vi "总磷氨氮插入数据.vi"(0 "database":string, 1 "data":T1 {"单位" items=["ug/L", "mg/L", "ppm", "mg/m3", "cm", "ppb", "ug/m3", "%", "nmol/mol", "umol/mol", "MPN/L", "MPN/100ml", "ng/m3", "NTU", "无量纲", "ms/cm", "us/cm"]}, 3 "SN":string, 5 "table":string, 7 "测量模式":T2(ring)=enum."水样测试", 9 "数据标记表":string(combo)="N", 11 "error in (no error)":errorcluster) -> (15 "error out":errorcluster)   [LabVIEW 2016, in "斯坦道氨氮.lvlib"]
uses:
  <vilib>/Utility/sysdir.llb/System Directory Type.ctl
  <vilib>/Utility/error.llb/DialogType.ctl
  <vilib>/addons/database/Connection.llb/DB Tools Open Connec (String).vi
  <vilib>/addons/database/Connection.llb/Conn Execute.vi
  <vilib>/addons/database/Recordset.llb/Rec Destroy - Connection.vi
  <vilib>/addons/database/Recordset.llb/Rec Fetch Recordset Data (R).vi
  <vilib>/addons/database/NI_Database_API.lvlib
panel:
  out "为空？":bool
  out "recordset data":variant[][](array[variant])
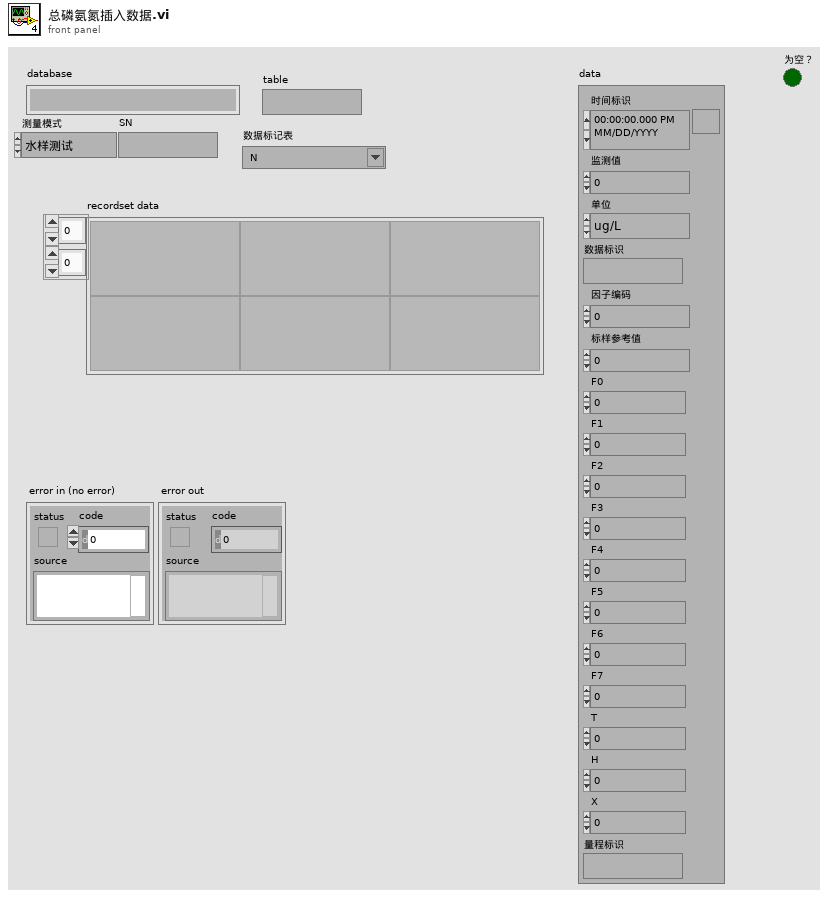
[diagram p1: front panel]
types:
  T1 = cluster{"时间标识":timestamp, "监测值":sgl, "单位":u16, "数据标识":string, "因子编码":u32, "标样参考值":sgl, "F0":sgl, "F1":sgl, "F2":sgl, "F3":sgl, "F4":sgl, "F5":sgl, "F6":sgl, "F7":sgl, "T":sgl, "H":sgl, "X":sgl, "量程标识":string}
  T2 = enum16{"维护数据", "水样测试", "标样核查", "零点核查", "跨度核查", "空白测试", "平行样测试", "加标回收", "空白校准", "标样校准", "初始化（清洗）"}
  T3 = typedef "DialogType.ctl" = u16
  T4 = typedef "System Directory Type.ctl" = i32
  T5 = typedef "NI_Database_API.lvlib/Conn ObjectReference.ctl" = refnum<k1>
  T6 = typedef "NI_Database_API.lvlib/Rec ObjectReference.ctl" = refnum<k1>
  T7 = cluster{"时间标识":timestamp, "测量模式":string, "数据类型":string, "监测值":sgl, "单位":string, "数据标识":string, "因子编码":string, "标样参考值":sgl, "F0":sgl, "F1":sgl, "F2":sgl, "F3":sgl, "F4":sgl, "F5":sgl, "F6":sgl, "F7":sgl, "温度":sgl, "湿度":sgl, "X":sgl, "量程标识":string, "SN":string, "LastTime":timestamp}
  T8 = cluster{"时间标识":timestamp, "设备":string, "日志信息":string}
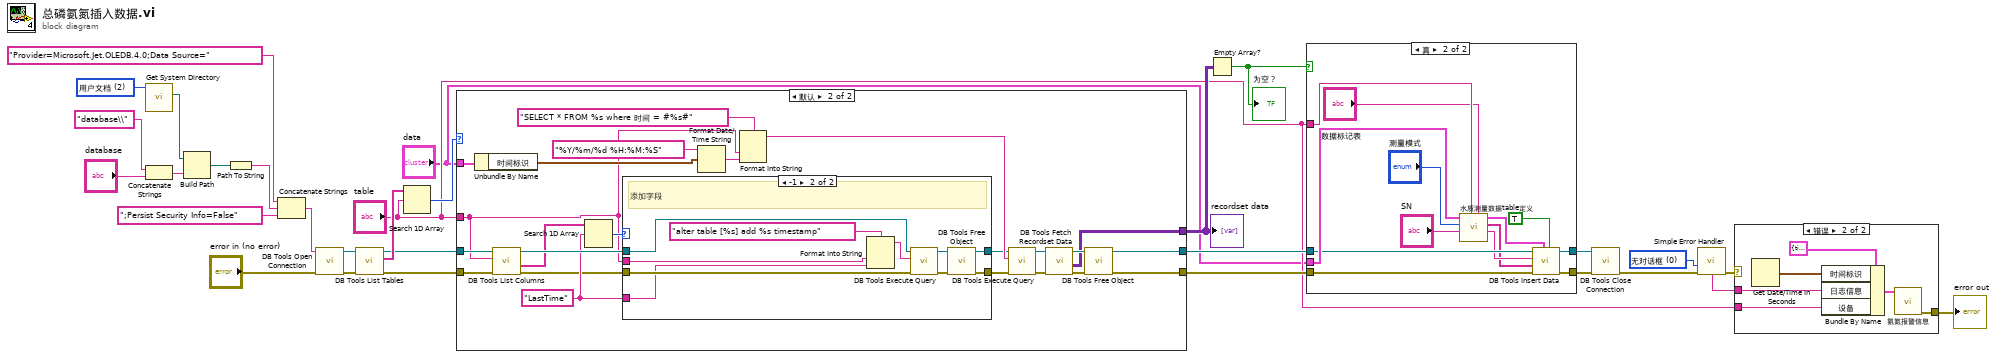
[diagram p0: block diagram]
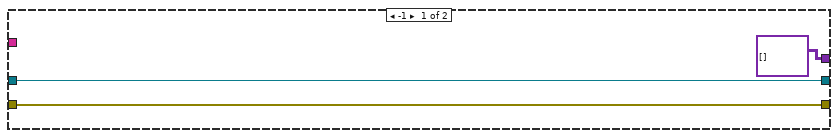
[diagram p3: hidden frame]
diagram:
  w6 = T3 0 items=["无对话框", "确定信息", "继续或停止信息", "确定信息＋警告", "继续/停止+警告"] ("type of dialog (OK msg:1)")
  w29 = T4 2 items=["用户目录"=0, "用户桌面"=1, "用户文档"=2, "用户应用程序数据"=3, "用户设置"=4, "用户临时目录"=5, "公共文档"=6, "公共应用程序数据"=7, "公共设置"=8, "公共缓存"=13, "系统核心库"=9, "系统安装库"=10, "应用程序文件"=11, "启动盘根目录"=12] ("system directory type")
  n1 = call <vilib>:"Get System Directory.vi"("system directory type"=w29) -> ("system directory"=w27:path)  [unwired: 10 in]
  n2 = Concatenate Strings("database\\" ("condition"), "database") -> (w21:string)
  n3 = Build Path(base path=w27, name or relative path=w21) -> (appended path=w26:path)
  n4 = Path To String(path=w26) -> (string=w25:string)
  n5 = Concatenate Strings("Provider=Microsoft.Jet.OLEDB.4.0;Data Source=" ("condition"), w25, ";Persist Security Info=False" ("condition")) -> (w23:string)
  n6 = call-poly <vilib>:"DB Tools Open Connection.vi"("error in (no error)"="error in (no error)", "connection information"=w23) -> ("error out"=w19:errorcluster, "connection reference"=w20:T5)  [unwired: 6 in]
  n7 = call <vilib>:"DB Tools List Tables.vi"("error in (no error)"=w19, "connection reference"=w20) -> ("error out"=w11:errorcluster, "tables"=w18:string[], "connection reference out"=w12:T5)  [unwired: 3 in]
  n8 = Search 1D Array(1D array=w18, element="table") -> (index of element=w13:i32)  [unwired: 1 in]
  n9 = case shown="默认" w13 {
    tunnel: [variant[][] [] ("recordset data") w36] -> w10
    tunnel: [w33 w52] -> w9
    tunnel: [w32 w51] -> w8
    tunnel: w12 -> [w33 w38]
    tunnel: w11 -> [w32 w37]
    tunnel: "table" -> [_ w35]
    tunnel: "data" -> [_ w46]
    frame -1 {
    }
    frame Default {
      w44 = "LastTime" ("元素")
      n10 = Unbundle By Name(w46) -> ("时间标识"=w49:timestamp)
      n11 = call <vilib>:"DB Tools List Columns.vi"("error in (no error)"=w37, "table"=w35, "connection reference"=w38) -> ("error out"=w42:errorcluster, "columns"=w43:string[], "connection reference out"=w45:T5)  [unwired: 1 in, 1 out]
      n12 = Search 1D Array(1D array=w43, element=w44) -> (index of element=w41:i32)  [unwired: 1 in]
      n13 = case shown="-1" w41 {
        tunnel: w45 -> [w58 w66]
        tunnel: w42 -> [w57 w65]
        tunnel: w44 -> [_ w63]
        tunnel: [w58 w61] -> w40
        tunnel: [w57 w60] -> w39
        tunnel: w35 -> [_ w59]
        frame 0, Default {
        }
        frame -1 {
          # "添加字段"
          n14 = Format Into String(format string="alter table [%s] add %s timestamp", w59, w63) -> (resulting string=w62:string)  [unwired: 2 in, 1 out]
          n15 = call-poly <vilib>:"DB Tools Execute Query.vi"("error in (no error)"=w65, "SQL query"=w62, "connection reference"=w66) -> ("error out"=w67:errorcluster, "recordset reference"=w68:T6)  [unwired: 5 in]
          n16 = call-poly <vilib>:"DB Tools Free Object.vi"("error in (no error)"=w67, "recordset reference"=w68) -> ("error out"=w60:errorcluster, "connection reference"=w61:T5)  [unwired: 8 in]
        }
      }
      n17 = Format Date/Time String(time format string (%c)="%Y/%m/%d %H:%M:%S" ("时间格式字符串(%c)"), seconds (now)=w49) -> (date/time string=w47:string)  [unwired: 1 in]
      n18 = Format Into String(format string="SELECT * FROM %s where 时间 = #%s#" ("格式字符串"), w35, w47) -> (resulting string=w50:string)  [unwired: 2 in, 1 out]
      n19 = call-poly <vilib>:"DB Tools Execute Query.vi"("error in (no error)"=w39, "SQL query"=w50, "connection reference"=w40) -> ("error out"=w53:errorcluster, "recordset reference"=w56:T6)  [unwired: 5 in]
      n20 = call-poly <vilib>:"DB Tools Fetch Recordset Data.vi"("error in (no error)"=w53, "recordset reference"=w56) -> ("error out"=w54:errorcluster, "recordset data"=w36:variant[][], "recordset reference out"=w55:T6)  [unwired: 3 in]
      n21 = call-poly <vilib>:"DB Tools Free Object.vi"("error in (no error)"=w54, "recordset reference"=w55) -> ("error out"=w51:errorcluster, "connection reference"=w52:T5)  [unwired: 8 in]
    }
  }
  "recordset data" <- w10
  n22 = Empty Array?(array=w10) -> (empty?=w16:bool)
  "为空？" <- w16
  n23 = case shown="真" w16 {
    tunnel: "table" -> [_ w83]
    tunnel: "data" -> [_ w82]
    tunnel: w8 -> [w69 w80]
    tunnel: w9 -> [w70 w79]
    tunnel: [w70 w74] -> w15
    tunnel: [w69 w73] -> w14
    frame False {
    }
    frame True {
      n24 = call "水质测量数据table定义.vi"("数据标记表"="数据标记表", "table 输入"=w83, "SN"="SN", "测量模式"="测量模式", "data"=w82) -> ("table 输出"=w76:string, "columns"=w75:string[], "data输出"=w78:T7)  [unwired: 4 in]
      n25 = call <vilib>:"DB Tools Insert Data.vi"("create table? (F)"=TRUE, "data"=w78, "error in (no error)"=w80, "columns"=w75, "table"=w76, "connection reference"=w79) -> ("error out"=w73:errorcluster, "connection reference out"=w74:T5)  [unwired: 4 in]
    }
  }
  n26 = call <vilib>:"DB Tools Close Connection.vi"("error in (no error)"=w14, "connection reference"=w15) -> ("error out"=w7:errorcluster)  [unwired: 5 in]
  n27 = call <vilib>:"Simple Error Handler.vi"("type of dialog (OK msg:1)"=w6, "error in (no error)"=w7) -> ("error out"=w5:errorcluster, "message"=w4:string)  [unwired: 3 in, 3 out]
  n28 = case shown="错误" w5 {
    tunnel: w4 -> [_ w85]
    tunnel: [_ w87] -> w3
    tunnel: "table" -> [_ w84]
    frame No Error {
    }
    frame Error {
      n29 = Get Date/Time In Seconds() -> (seconds since 1Jan1904=w86:timestamp)
      n30 = Bundle By Name(cluster=T8 {"时间标识"=timestamp(0 s since 1904-01-01), "设备"="氨氮", "日志信息"=""} ("data in"), "时间标识"=w86, "日志信息"=w85, "设备"=w84) -> (w88:T8)
      n31 = call "氨氮报警信息.vi"("data in"=w88) -> ("error out"=w87:errorcluster)  [unwired: 10 in]
    }
  }
  "error out" <- w3
